vi "Close Sessions.vi"(8 "error in":errorcluster, 11 "session reservation in":refnum<class "Session Reservation.lvclass">) -> (0 "error out":errorcluster, 3 "session reservation out":refnum<class "Session Reservation.lvclass">)   [LabVIEW 2020, in "NI Session Management V1 Client.lvlib" / "Session Reservation.lvclass"]
doc: "Closes all instrument sessions that were created with the session reservation."
uses:
  Session Reservation.lvclass
  Session Reservation.lvclass/Session Reservation.ctl
  Sessions/Instrument/ISession Factory/ISession Factory.lvclass
  Measurements/Helpers/Error Strings Global Internal.vi
  <vilib>/Utility/error.llb/Error Cluster From Error Code.vi
  Connection Map/Connection Map.lvclass
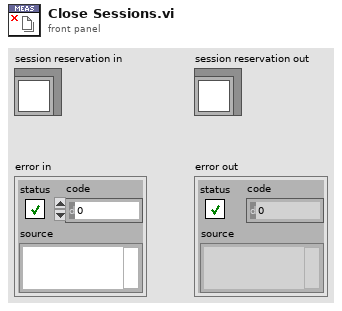
[diagram p1: front panel]
types:
  T1 = typedef "NI Session Management V1 Client.lvlib/Session Reservation.lvclass/Data.ctl" = cluster{"session and driver infos":T2[], "pin or relay names":string[], "connection map":refnum<class "Connection Map.lvclass">, "pin map context":T7, "reservation observer":refnum<class "IReservation Observer.lvclass">, "dvr valid":bool, "group mappings":T8}
  T2 = typedef "NI Session Management V1 Client.lvlib/Session Reservation.lvclass/Session and Driver Info.ctl" = cluster{"session info":T3, "session":variant, "session factory":refnum<class "ISession Factory.lvclass">, "initialize and close session behavior":T6}
  T3 = typedef "ni.measurementlink.sessionmanagement.v1.api.lvlib/ni_measurementlink_sessionmanagement_v1_SessionInformation.ctl" = cluster{"session":T4, "resource_name":string, "channel_list":string, "instrument_type_id":string, "session_exists":bool, "channel_mappings":T5[]}
  T4 = typedef "ni.measurementlink.sessionmanagement.v1.api.lvlib/nidevice_grpc_Session.ctl" = cluster{"name":string}
  T5 = typedef "ni.measurementlink.sessionmanagement.v1.api.lvlib/ni_measurementlink_sessionmanagement_v1_ChannelMapping.ctl" = cluster{"pin_or_relay_name":string, "site":i32, "channel":string, "multiplexer_resource_name":string, "multiplexer_route":string}
  T6 = typedef "NI Session Management Instrument.lvlib/ISession Factory.lvclass/Initialize and Close Session Behavior.ctl" = enum16{"Initialize and Close", "Attach and Detach", "Initialize and Detach", "Attach and Close"}
  T7 = typedef "ni.measurementlink.sessionmanagement.v1.api.lvlib/ni_measurementlink_PinMapContext.ctl" = cluster{"pin_map_id":string, "sites":i32[]}
  T8 = typedef "NI Session Management V1 Client.lvlib/Session Reservation.lvclass/Group Mapping.ctl" = map{string, string[]}
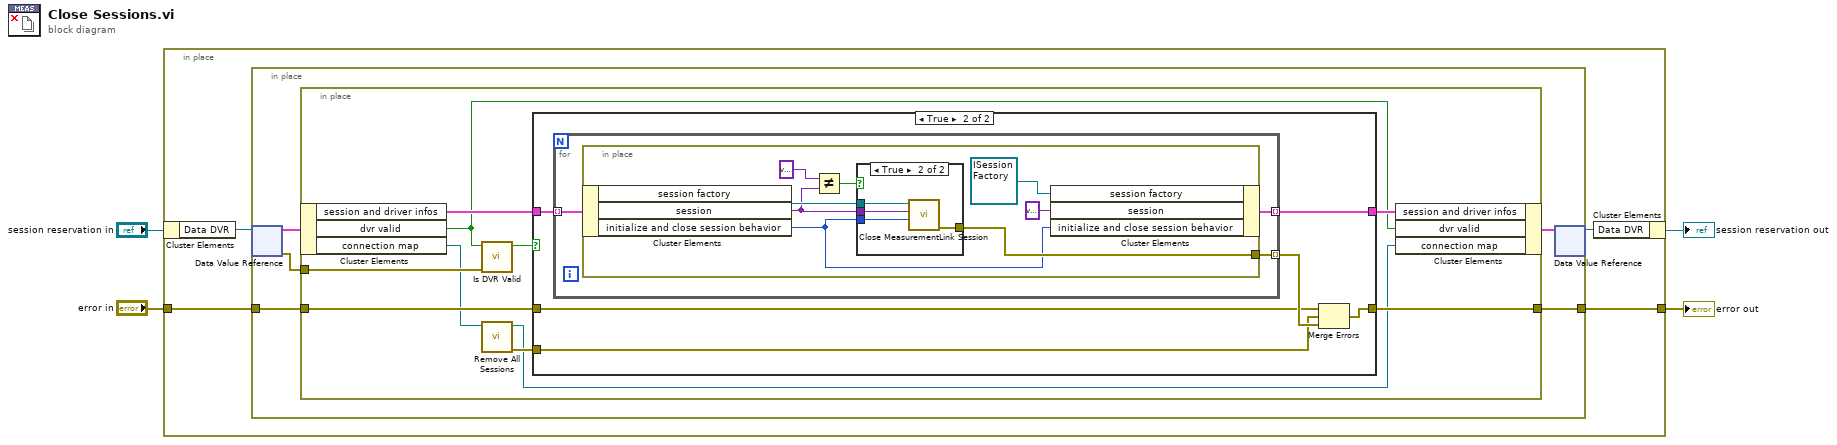
[diagram p0: block diagram]
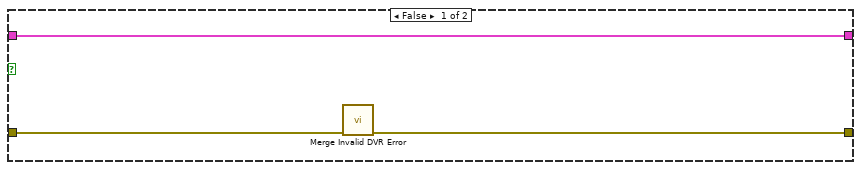
[diagram p2: hidden frame]
diagram:
  n1 = in-place {
    in-place-border: [w6] -> w1
    in-place-border: "error in" -> [w5]
    n2 = in-place-cluster #1("session reservation in") -> ("Data DVR"=w8:refnum<data-value>)
    n3 = in-place {
      in-place-border: [w10] -> w6
      in-place-border: w5 -> [w11]
      n4 = in-place-dvr #2(w8) -> (w12:T1, w13:errorcluster)
      n5 = in-place {
        in-place-border: w13 -> [w23]
        in-place-border: w11 -> [w18]
        in-place-border: [w17] -> w10
        n6 = in-place-cluster #3(w12) -> ("session and driver infos"=w21:T2[], "dvr valid"=w19:bool, "connection map"=w15:refnum<class "Connection Map.lvclass">)
        n7 = call "Is DVR Valid.vi"("dvr error in"=w23, "dvr valid in"=w19) -> ("dvr valid out"=w22:bool)  [unwired: 9 in]
        n8 = call "Remove All Sessions.vi"("connection map in"=w15) -> ("error out"=w16:errorcluster, "connection map out"=w14:refnum<class "Connection Map.lvclass">)  [unwired: 9 in]
        n9 = case shown="True" w22 {
          tunnel: w21 -> [w26 w32]
          tunnel: [w26 w31] -> w20
          tunnel: w18 -> [w25 w27]
          tunnel: [w24 w30] -> w17
          tunnel: w16 -> [_ w28]
          frame False {
            n10 = call "Merge Invalid DVR Error.vi"("error in"=w25) -> ("error out"=w24:errorcluster)  [unwired: 10 in]
          }
          frame True {
            n11 = for {
              tunnel: w32 -> [w35] mode=indexing
              tunnel: [w34] -> w31 mode=indexing
              tunnel: [w33] -> w29 mode=indexing
              n12 = in-place {
                in-place-border: [w42] -> w33
                n13 = in-place-cluster #4(w35) -> ("session factory"=w41:refnum<class "ISession Factory.lvclass">, "session"=w37:variant, "initialize and close session behavior"=w39:T6)
                n14 = Not Equal?(x=variant, y=w37) -> (x != y?=w38:bool)
                n15 = case shown="True" w38 {
                  tunnel: w37 -> [_ w47]
                  tunnel: [_ w46] -> w42
                  tunnel: w41 -> [_ w45]
                  tunnel: w39 -> [_ w44]
                  frame False {
                  }
                  frame True {
                    n16 = call-dynamic "Close MeasurementLink Session.vi"("initialize and close session behavior"=w44, "session in"=w47, "session factory in"=w45) -> ("error out"=w46:errorcluster)  [unwired: 8 in]
                  }
                }
                n17 = in-place-cluster #4("session factory"=refnum<class "ISession Factory.lvclass"> refnum ("instrument"), "session"=variant, "initialize and close session behavior"=w39) -> (w34:T2)
              }
            }
            n18 = Merge Errors(w27, w28, w29) -> (w30:errorcluster)
          }
        }
        n19 = in-place-cluster #3("session and driver infos"=w20, "dvr valid"=w19, "connection map"=w14) -> (w9:T1)
      }
      n20 = in-place-dvr #2(w9) -> (w7:refnum<data-value>)  [unwired: 1 out]
    }
    n21 = in-place-cluster #1("Data DVR"=w7) -> (→"session reservation out":refnum<class "Session Reservation.lvclass">)
  }
  "error out" <- w1
